vi "Pre Launch Init.vi"(11 "DMM Driver in":refnum<class "DMM Driver.lvclass">) -> (0 "error out":errorcluster, 3 "DMM Driver out":refnum<class "DMM Driver.lvclass">)   [LabVIEW 2020, in "DMM Driver.lvclass"]
doc: "(<B>Filename</B>: Actor Framework.lvlib:Actor.lvclass:Pre Launch Init.vi)\n\nDefines behavior that occurs after the Launch Actor method is invoked but before the actor's Actor Core method begins running.\n\nThe Pre Launch Init method is guaranteed to finish before the Launch Actor method returns to its caller and before the actor itself receives any messages. Any references that the Pre Launch Init method obtains are guaranteed to have the same lifetime as the actor itself. Any errors that the Pre Launch Init method returns will abort the launch.\n\nBy default, this method does nothing. A descendant class may override it to define behavior."
uses:
  DMM Driver.lvclass
  DMM/DMM.lvclass
  DMM Driver.lvclass/DMM Driver.ctl
  <vilib>/ActorFramework/Actor/Actor.lvclass
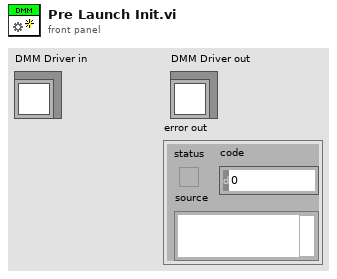
[diagram p1: front panel]
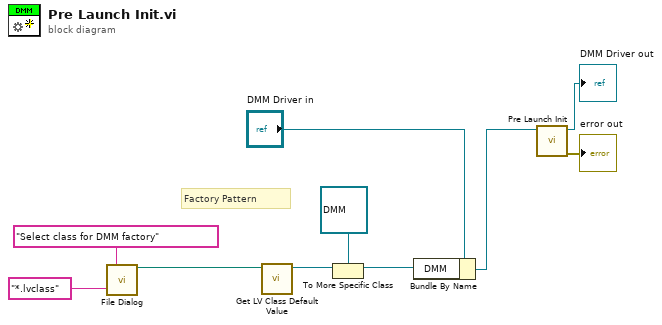
[diagram p0: block diagram]
diagram:
  # "Factory Pattern"
  n1 = call "File Dialog"("prompt"="Select class for DMM factory", "pattern (all files)"="*.lvclass") -> ("selected path"=w3:path)  [unwired: 10 in, 3 out]
  n2 = call <vilib>:"Get LV Class Default Value.vi"("class path"=w3) -> ("object"=w8:refnum<class>)  [unwired: 9 in, 1 out]
  n3 = To More Specific Class(target class=refnum<class "DMM.lvclass"> refnum ("DMM.lvclass"), reference=w8) -> (specific class reference=w6:refnum<class "DMM.lvclass">)  [unwired: 1 in, 1 out]
  n4 = Bundle By Name(cluster="DMM Driver in", "DMM"=w6) -> (w4:refnum<class "DMM Driver.lvclass">)
  n5 = call-parent "Pre Launch Init.vi"("Actor in"=w4) -> ("error out"=→"error out":errorcluster, "Actor out"=→"DMM Driver out":refnum<class "DMM Driver.lvclass">)  [unwired: 9 in]
